vi "Read Identifier.vi"(8 "error in (no error)":errorcluster, 11 "CAN Communicator in":refnum<class "Oil.lvclass">) -> (0 "error out":errorcluster, 2 "identifier":u32=523 format="%x", 3 "CAN Communicator out":refnum<class "Oil.lvclass">)   [LabVIEW 2015, in "Oil.lvclass"]
uses:
  Oil.lvclass
  Oil.lvclass/Oil.ctl
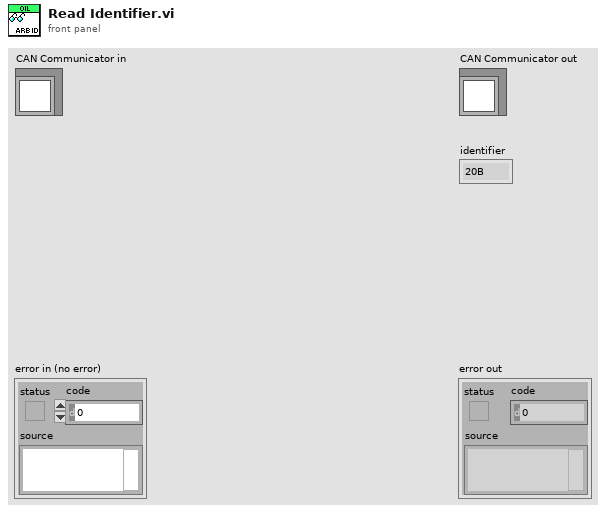
[diagram p1: front panel]
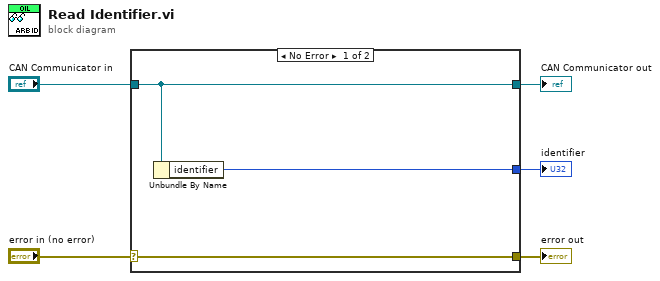
[diagram p0: block diagram]
diagram:
  n1 = case shown="No Error" "error in (no error)" {
    selector: "error in (no error)" -> [w8 w9]
    tunnel: [w8 w9] -> w4
    tunnel: [w7 w10] -> w2
    tunnel: "CAN Communicator in" -> [w7 w10]
    tunnel: [w6 _] -> w1
    frame No Error {
      n2 = Unbundle By Name(w7) -> ("identifier"=w6:u32)
    }
    frame Error {
    }
  }
  "error out" <- w4
  "CAN Communicator out" <- w2
  "identifier" <- w1
